vi "Expand Training Data.vi"() -> ()   [LabVIEW 2021]
uses:
  <vilib>/Utility/file.llb/Read Delimited Spreadsheet (DBL).vi
  <vilib>/Utility/file.llb/Write Delimited Spreadsheet (DBL).vi
panel:
  out "Success":bool
  in  "CSV to be merged":path
  in  "Original CSV":path
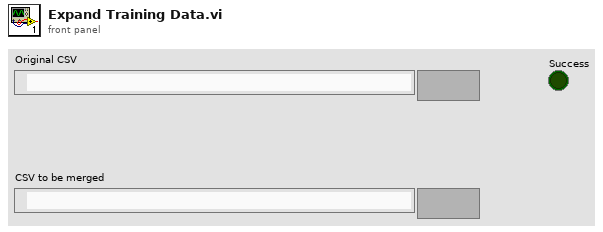
[diagram p1: front panel]
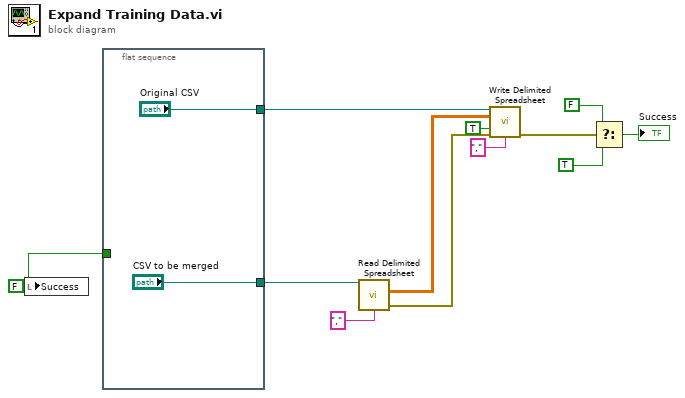
[diagram p0: block diagram]
diagram:
  w2 = FALSE ("s? t:f")
  n1 = local write "Success"(w2) -> ()
  n2 = flat-sequence {
    tunnel: ["Original CSV"] -> w12
    tunnel: ["CSV to be merged"] -> w9
    tunnel: w2 -> [_]
    frame #0 {
    }
  }
  n3 = call-poly <vilib>:"Read Delimited Spreadsheet.vi"("file path (dialog if empty)"=w9, "delimiter (\\t)"="," ("delimiter (\\t)")) -> ("all rows"=w7:dbl[][], "error out"=w1:errorcluster)  [unwired: 8 in, 4 out]
  n4 = call-poly <vilib>:"Write Delimited Spreadsheet.vi"("file path (dialog if empty)"=w12, "2D data"=w7, "append to file? (new file:F)"=TRUE, "error in (no error)"=w1, "delimiter (\\t)"="," ("delimiter (\\t)")) -> ("error out"=w6:errorcluster)  [unwired: 9 in, 1 out]
  n5 = Select(t=FALSE, s=w6, f=TRUE) -> (s? t:f=→"Success":bool)
